vi "acc_gyro_enc to waveform.vi"(11 "acc gyro data":T1) -> (1 "encoder":waveform(dbl), 2 "accel plot":waveform(dbl)[](array[waveform]), 3 "gyro plot":waveform(dbl)[](array[waveform]))   [LabVIEW 2012]
uses:
  acc_gyro_enc_data.ctl
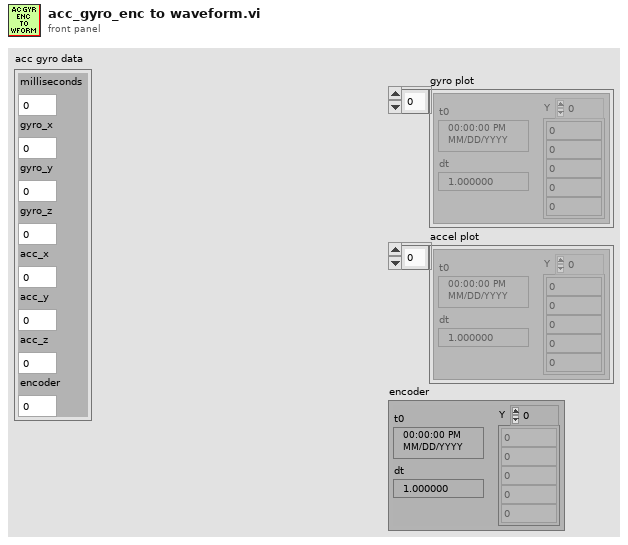
[diagram p1: front panel]
types:
  T1 = typedef "acc_gyro_enc_data.ctl" = cluster{"milliseconds":u64, "gyro_x":dbl, "gyro_y":dbl, "gyro_z":dbl, "acc_x":dbl, "acc_y":dbl, "acc_z":dbl, "encoder":dbl}
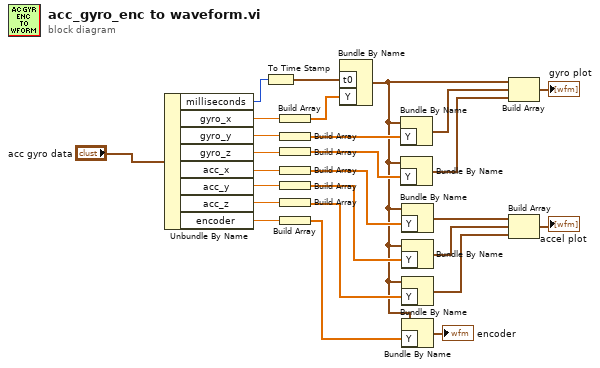
[diagram p0: block diagram]
diagram:
  n1 = Unbundle By Name("acc gyro data") -> ("milliseconds"=w25:u64, "gyro_x"=w23:dbl, "gyro_y"=w21:dbl, "gyro_z"=w20:dbl, "acc_x"=w19:dbl, "acc_y"=w18:dbl, "acc_z"=w17:dbl, "encoder"=w3:dbl)
  n2 = To Time Stamp(1:w25) -> (0:w24:timestamp)
  n3 = Build Array(w23) -> (w22:dbl[])
  n4 = Build Array(w21) -> (w16:dbl[])
  n5 = Build Array(w20) -> (w15:dbl[])
  n6 = Build Array(w19) -> (w14:dbl[])
  n7 = Build Array(w18) -> (w13:dbl[])
  n8 = Build Array(w17) -> (w12:dbl[])
  n9 = Build Array(w3) -> (w2:dbl[])
  n10 = Bundle By Name("t0"=w24, "Y"=w22) -> (w4:waveform(dbl))  [unwired: 1 in]
  n11 = Bundle By Name(cluster=w4, "Y"=w16) -> (w11:waveform(dbl))
  n12 = Bundle By Name(cluster=w4, "Y"=w15) -> (w10:waveform(dbl))
  n13 = Bundle By Name(cluster=w4, "Y"=w14) -> (w9:waveform(dbl))
  n14 = Bundle By Name(cluster=w4, "Y"=w13) -> (w8:waveform(dbl))
  n15 = Bundle By Name(cluster=w4, "Y"=w12) -> (w7:waveform(dbl))
  n16 = Bundle By Name(cluster=w4, "Y"=w2) -> (→"encoder":waveform(dbl))
  n17 = Build Array(w4, w11, w10) -> (→"gyro plot":waveform(dbl)[])
  n18 = Build Array(w9, w8, w7) -> (→"accel plot":waveform(dbl)[])
